vi "Read Type.vi"(8 "error in (no error)":errorcluster, 11 "Data2D in":refnum<class "Data2D.lvclass">) -> (0 "error out":errorcluster, 2 "Type":string, 3 "Data2D out":refnum<class "Data2D.lvclass">)   [LabVIEW 2018, in "Data2D.lvclass"]
uses:
  Data2D.lvclass
  Data2D.lvclass/Data2D.ctl
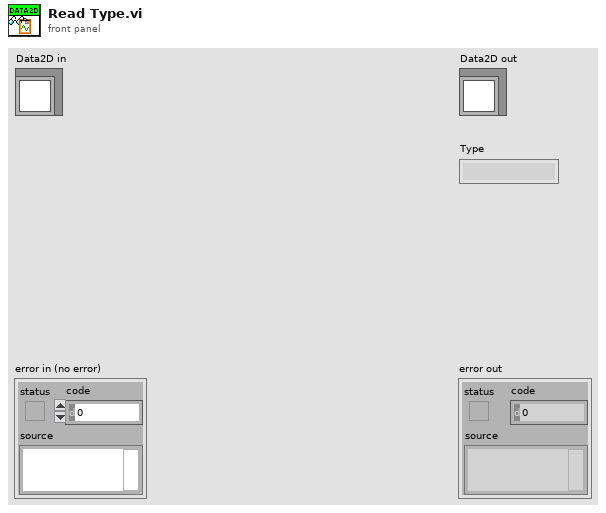
[diagram p1: front panel]
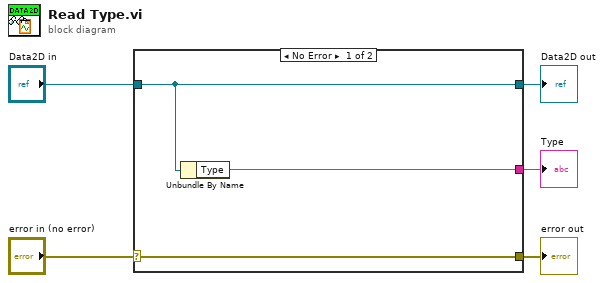
[diagram p0: block diagram]
diagram:
  n1 = case shown="No Error" "error in (no error)" {
    selector: "error in (no error)" -> [w8 w9]
    tunnel: [w8 w9] -> w4
    tunnel: [w7 w10] -> w2
    tunnel: "Data2D in" -> [w7 w10]
    tunnel: [w6 _] -> w1
    frame No Error {
      n2 = Unbundle By Name(w7) -> ("Type"=w6:string)
    }
    frame Error {
    }
  }
  "error out" <- w4
  "Data2D out" <- w2
  "Type" <- w1
